vi "createtable.vi"(8 "CalData":string[][](array[string])) -> (0 "tab output":string)   [LabVIEW 2012]
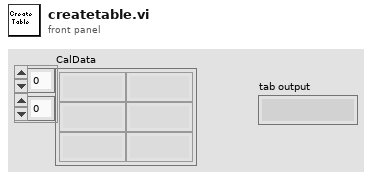
[diagram p1: front panel]
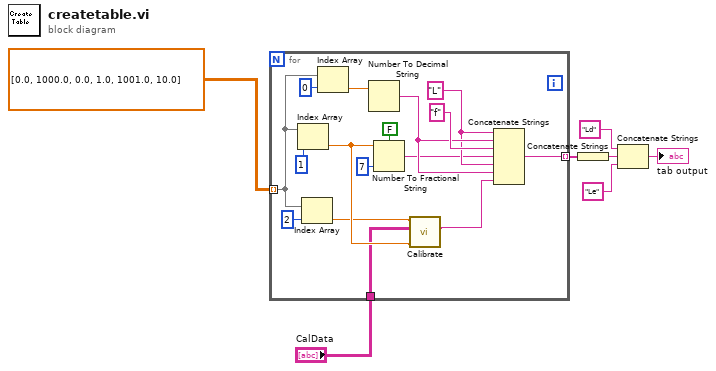
[diagram p0: block diagram]
diagram:
  n1 = for {
    tunnel: dbl[][] [[0.0, 1000.0, 0.0], [1.0, 1001.0, 10.0]] ("Sweep Table") -> [w12] mode=indexing
    tunnel: [w18] -> w4 mode=indexing
    tunnel: "CalData" -> [w8]
    w15 = "L" ("string")
    n2 = Index Array(array=w12, index=1) -> (element=w10:dbl)
    n3 = Index Array(array=w12, index=2) -> (element=w9:dbl)
    n4 = Index Array(array=w12, index=0) -> (element=w16:dbl)
    n5 = Number To Decimal String(number=w16) -> (decimal integer string=w19:string)  [unwired: 1 in]
    n6 = Number To Fractional String(use system decimal point (T)=FALSE, number=w10, precision (6)=i16 7) -> (F-format string=w14:string)  [unwired: 1 in]
    n7 = call "Calibrate.vi"("RF  FREQUENCY MHz"=w10, "CalData"=w8, "RF Power In"=w9) -> ("cal level"=w11:string)  [unwired: 6 in, 2 out]
    n8 = Concatenate Strings(w15, w19, "f" ("string"), w14, w15, w19, w11) -> (w18:string)
  }
  n9 = Concatenate Strings(w4) -> (w6:string)
  n10 = Concatenate Strings("Ld" ("string"), w6, "Le" ("string")) -> (→"tab output":string)
